vi "PruebaSeq.vi"() -> ()   [LabVIEW 2014, in "MSX-E3701_dll.lvlib"]
uses:
  MSX-E3701_dll.lvlib
  Typedef/Config Data.ctl
  Typedef/Connection Data.ctl
  E:/Repositorio Magnis/INF002/v0/Modules/HAL/Drivers/Sync/ADDI-DATA MSX-E3701/API/MX370x.dll
  MX370x.dll
  E:/Repositorio Magnis/INF002/v0/Modules/HAL/Drivers/Sync/ADDI-DATA MSX-E3701/API/MXCommon.dll
  MXCommon.dll
  Typedef/Adquisition Data.ctl
panel:
  in  "stop 2":bool
  out "Waveform Chart":u32[][](graph)
  in  "stop":bool
  out "Adquisition Data":T1
  out "error out":errorcluster
  in  "Connection Data In":T2
  in  "Error In":errorcluster
  in  "Config Data":T3
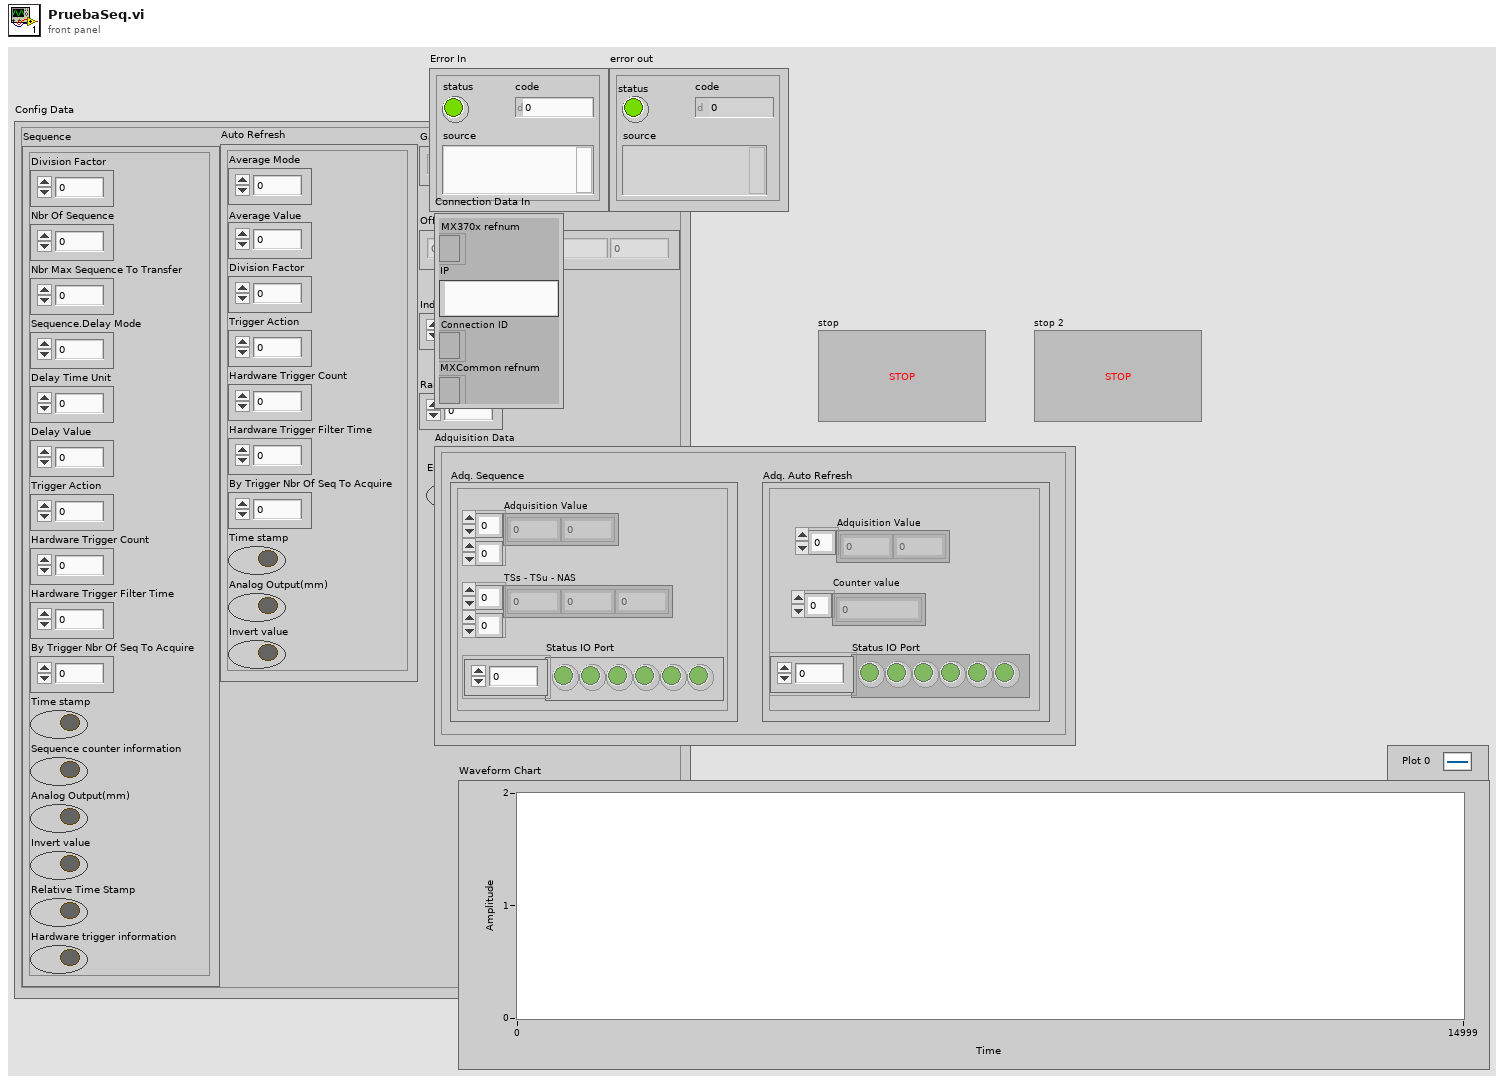
[diagram p1: front panel]
types:
  T1 = typedef "MSX-E3701_dll.lvlib/Adquisition Data.ctl" = cluster{"Adq. Sequence":cluster{"TSs - TSu - NAS":u64[][], "Adquisition Value":u32[][], "Status IO Port":bool[]}, "Adq. Auto Refresh":cluster{"Adquisition Value":u64[], "Status IO Port":bool[], "Counter value":u64[]}}
  T2 = typedef "MSX-E3701_dll.lvlib/Connection Data.ctl" = cluster{"MX370x refnum":refnum<k24>, "IP":string, "Connection ID ":refnum<k5>, "MXCommon refnum":refnum<k24>}
  T3 = typedef "MSX-E3701_dll.lvlib/Config Data.ctl" = cluster{"Auto Refresh":cluster{"Average Mode":u64, "Average Value":u64, "Division Factor":u64, "Trigger Action":u64, "Hardware Trigger Count":u64, "Hardware Trigger Filter Time":u64, "By Trigger Nbr Of Seq To Acquire":u64, "Time stamp":bool, "Analog Output(mm)":bool, "Invert value":bool}, "Gain":sgl[], "Offset":sgl[], "Index":u64, "Range":sgl, "Sequence":cluster{"Division Factor":u64, "Nbr Of Sequence":u64, "Nbr Max Sequence To Transfer":u64, "Sequence.Delay Mode":u64, "Delay Time Unit":u64, "Delay Value":u64, "Trigger Action":u64, "Hardware Trigger Count":u64, "Hardware Trigger Filter Time":u64, "By Trigger Nbr Of Seq To Acquire":u64, "Time stamp":bool, "Sequence counter information":bool, "Analog Output(mm)":bool, "Invert value":bool, "Relative Time Stamp":bool, "Hardware trigger information":bool}, "Enable DIO":bool}
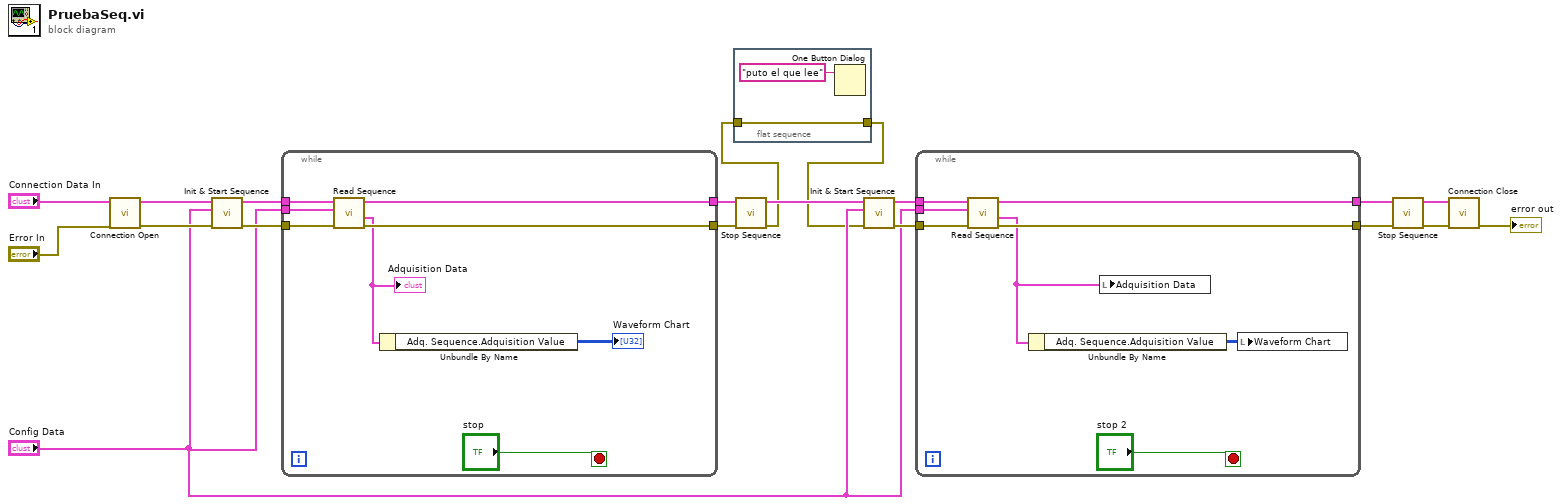
[diagram p0: block diagram]
diagram:
  n1 = call "Connection Open.vi"("Error In"="Error In", "Connection Data In"="Connection Data In") -> ("Error Out"=w18:errorcluster, "Connection Data Out"=w19:T2)  [unwired: 8 in]
  n2 = call "Init & Start Sequence.vi"("error in (no error)"=w18, "Config Data"="Config Data", "Connection Data In"=w19) -> ("error out"=w12:errorcluster, "Connection Data Out"=w14:T2)  [unwired: 7 in]
  n3 = while {
    tunnel: "Config Data" -> [w23]
    tunnel: w14 -> [w27]
    tunnel: [w26] -> w13
    tunnel: w12 -> [w25]
    tunnel: [w24] -> w11
    stop <- "stop" stop-if-true
    n4 = call "Read Sequence.vi"("error in (no error)"=w25, "Config Data"=w23, "Connection Data In"=w27) -> ("error out"=w24:errorcluster, "Adquisition Data Out"=w21:T1, "Connection Data Out"=w26:T2)  [unwired: 6 in]
    "Adquisition Data" <- w21
    n5 = Unbundle By Name(w21) -> ("Adq. Sequence.Adquisition Value"=→"Waveform Chart":u32[][])
  }
  n6 = flat-sequence {
    tunnel: [w28] -> w2
    tunnel: w1 -> [w28]
    frame #0 {
      n7 = One Button Dialog(message="puto el que lee") -> ()  [unwired: 1 in, 1 out]
    }
  }
  n8 = call "Stop Sequence.vi"("error in (no error)"=w11, "Connection Data In"=w13) -> ("error out"=w1:errorcluster, "Connection Data Out"=w6:T2)  [unwired: 8 in]
  n9 = call "Init & Start Sequence.vi"("error in (no error)"=w2, "Config Data"="Config Data", "Connection Data In"=w6) -> ("error out"=w4:errorcluster, "Connection Data Out"=w5:T2)  [unwired: 7 in]
  n10 = while {
    tunnel: "Config Data" -> [w33]
    tunnel: w5 -> [w37]
    tunnel: [w36] -> w9
    tunnel: w4 -> [w35]
    tunnel: [w34] -> w10
    stop <- "stop 2" stop-if-true
    n11 = call "Read Sequence.vi"("error in (no error)"=w35, "Config Data"=w33, "Connection Data In"=w37) -> ("error out"=w34:errorcluster, "Adquisition Data Out"=w30:T1, "Connection Data Out"=w36:T2)  [unwired: 6 in]
    n12 = Unbundle By Name(w30) -> ("Adq. Sequence.Adquisition Value"=w31:u32[][])
    n13 = local write "Adquisition Data"(w30) -> ()
    n14 = local write "Waveform Chart"(w31) -> ()
  }
  n15 = call "Stop Sequence.vi"("error in (no error)"=w10, "Connection Data In"=w9) -> ("error out"=w8:errorcluster, "Connection Data Out"=w7:T2)  [unwired: 8 in]
  n16 = call "Connection Close.vi"("error in (no error)"=w8, "Connection Data In"=w7) -> ("error out"=→"error out":errorcluster)  [unwired: 8 in, 1 out]
